vi "Add Implementation Child Tree.vi"(8 "error in":errorcluster, 11 "Data in":T1) -> (0 "error out":errorcluster, 3 "Data out":T1)   [LabVIEW 2020, in "Peek Window.lvlib"]
uses:
  Peek Window.lvlib
  MHL Data Cluster.ctl
  Open Diagram Argument--cluster.ctl
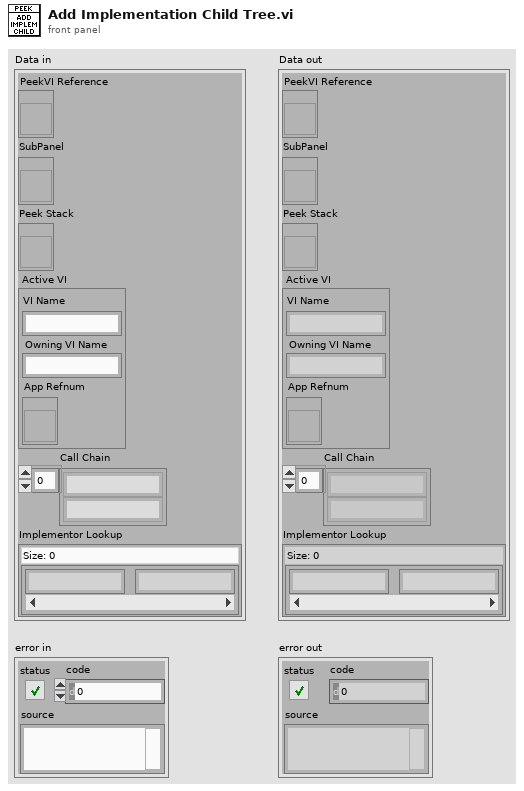
[diagram p1: front panel]
types:
  T1 = typedef "Peek Window.lvlib/MHL Data Cluster.ctl" = cluster{"PeekVI Reference":refnum<vi>, "SubPanel":refnum<vi>, "Peek Stack":refnum<vi>, "Active VI":T2, "Call Chain":string[], "Implementor Lookup":map{string, string}}
  T2 = typedef "Peek Window.lvlib/Open Diagram Argument--cluster.ctl" = cluster{"VI Name":string, "Owning VI Name":string, "App Refnum":refnum<vi>}
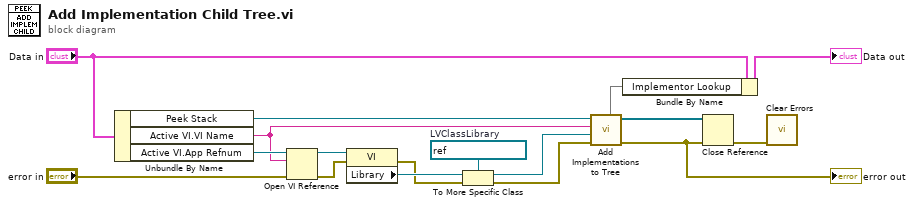
[diagram p0: block diagram]
diagram:
  w10 = refnum<vi> refnum  # LVClassLibrary
  n1 = Unbundle By Name("Data in") -> ("Peek Stack"=w17:refnum<vi>, "Active VI.VI Name"=w15:string, "Active VI.App Refnum"=w16:refnum<vi>)
  n2 = Open VI Reference(application reference (local)=w16, vi path=w15, error in (no error)="error in") -> (vi reference=w14:refnum<vi>, error out=w12:errorcluster)  [unwired: 3 in]
  n3 = property class="VI"(reference=w14, error in=w12) -> (error out=w9:errorcluster, "Library"=w13:refnum<vi>)  [unwired: 1 out]
  n4 = To More Specific Class(target class=w10, reference=w13, error in=w9) -> (specific class reference=w11:refnum<vi>, error out=w8:errorcluster)
  n5 = call "Add Implementations to Tree.vi"("error in (no error)"=w8, "Wired-in Class Refnum"=w11, "Method Name"=w15, "Tree Refnum"=w17) -> ("error out"=w5:errorcluster, "All Classes"=w1:refnum<vi>[], "Implementor Lookup"=w2:map{string, string})  [unwired: 4 in, 1 out]
  "error out" <- w5
  n6 = Bundle By Name(cluster="Data in", "Implementor Lookup"=w2) -> (→"Data out":T1)
  n7 = Close Reference(reference=w1, error in (no error)=w5) -> (error out=w6:errorcluster)
  n8 = call <vilib>:"Clear Errors.vi"("error in (no error)"=w6) -> ()  [unwired: 5 in, 2 out]
